vi "tipoPrueba.vi"() -> (0 "tipoPrueba":string)   [LabVIEW 2019, in "Prueba06.lvclass"]
uses:
  Prueba06.lvclass
panel:
  in  "inferior":bool
  in  "superior":bool
  # "¿Qué tipo de Prueba realizará?"
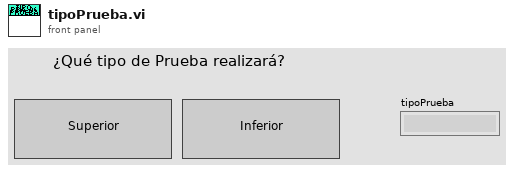
[diagram p1: front panel]
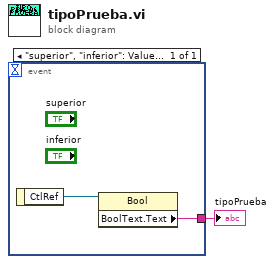
[diagram p0: block diagram]
diagram:
  n1 = event shown="[0] \"superior\", \"inferior\": Value Change" {
    selector: _ -> [_]
    dyn-events: _ -> [_]
    timeout: _ -> [_]
    tunnel: [w2] -> w1
    event "superior", "inferior": Value Change {
      n2 = event-data() -> ("CtlRef"=w3:refnum<vi>)  [unwired: 1 in]
      n3 = property class="Bool"(reference=w3) -> ("BoolText.Text"=w2:string)  [unwired: 1 in, 2 out]
    }
  }
  "tipoPrueba" <- w1
